vi "Load Users.json String.vi"(8 "error in (no error)":errorcluster) -> (0 "error out":errorcluster, 3 "Users Array":T1(array[cluster]))   [LabVIEW 2026, in "Local File Auth Provider.lvclass"]
uses:
  Local File Auth Provider.lvclass
  Local File Auth Provider.lvclass/Local File Auth Provider.ctl
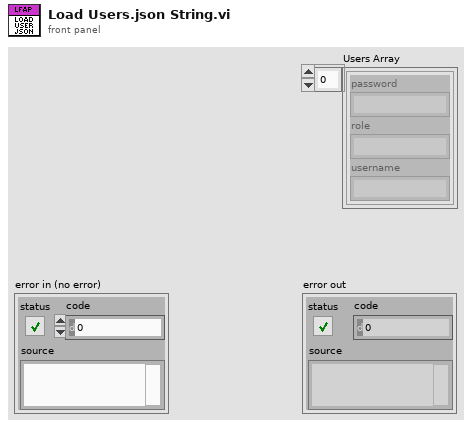
[diagram p1: front panel]
types:
  T1 = cluster{"password":string, "role":string, "username":string}[]
  T2 = cluster{"password":string, "role":string, "username":string}
  T3 = enum16{"open", "replace", "create", "open or create", "replace or create", "replace or create with confirmation"}
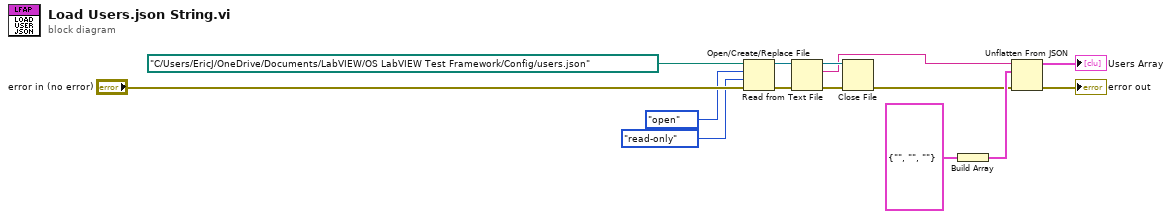
[diagram p0: block diagram]
diagram:
  n1 = Open/Create/Replace File(file path (use dialog)=path "C:/Users/EricJ/OneDrive/Documents/LabVIEW/OS LabVIEW Test Framework/Config/users.json" ("path to users.json"), error in="error in (no error)", operation (0:open)=T3."open", access (0:read/write)=enum16{"read/write", "read-only", "write-only"}."read-only") -> (refnum out=w7:refnum<file>, error out=w10:errorcluster)  [unwired: 2 in, 1 out]
  n2 = Read from Text File(file (use dialog)=w7, error in=w10) -> (refnum out=w11:refnum<file>, text=w2:string, error out=w12:errorcluster)  [unwired: 2 in, 1 out]
  n3 = Close File(refnum=w11, error in=w12) -> (error out=w4:errorcluster)  [unwired: 1 out]
  n4 = Build Array(T2 {"password"="", "role"="", "username"=""}) -> (w5:T1)
  n5 = Unflatten From JSON(JSON string=w2, type and defaults=w5, error in (no error)=w4) -> (value=→"Users Array":T1, error out=→"error out":errorcluster)  [unwired: 4 in]
